vi "Write SSL Context.vi"(8 "error in (no error)":errorcluster, 10 "SSL_Lib.lvlib:SSL-Context.lvclass":refnum<class "SSL-Context.lvclass">, 11 "SSL Context in":refnum<class "SSL Context.lvclass">) -> (0 "error out":errorcluster, 3 "SSL Context out":refnum<class "SSL Context.lvclass">)   [LabVIEW 2013, in "OpenSSL Socket.lvlib" / "SSL Context.lvclass"]
uses:
  SSL Context.lvclass
  SSL_Lib/SSL-Context/SSL-Context.lvclass
  SSL Context.lvclass/SSL Context.ctl
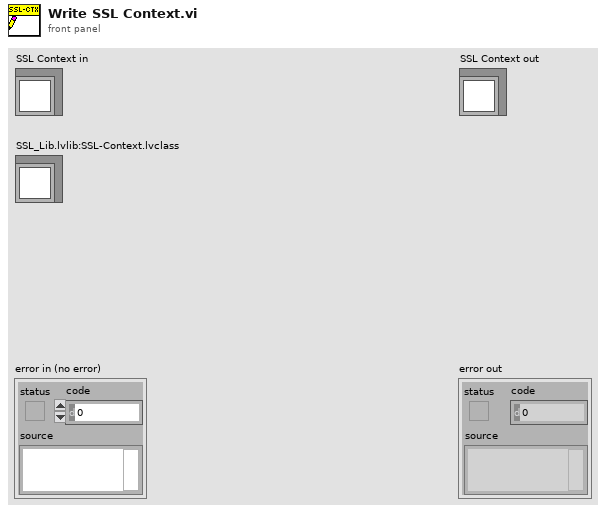
[diagram p1: front panel]
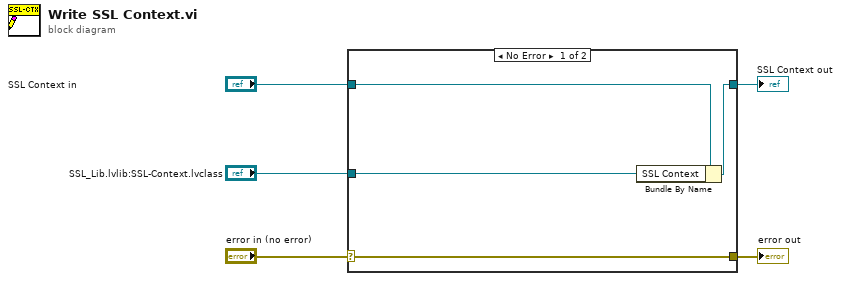
[diagram p0: block diagram]
diagram:
  n1 = case shown="No Error" "error in (no error)" {
    selector: "error in (no error)" -> [w9 w10]
    tunnel: [w9 w10] -> w4
    tunnel: [w7 w11] -> w2
    tunnel: "SSL Context in" -> [w8 w11]
    tunnel: "SSL_Lib.lvlib:SSL-Context.lvclass" -> [w6 _]
    frame No Error {
      n2 = Bundle By Name(cluster=w8, "SSL Context"=w6) -> (w7:refnum<class "SSL Context.lvclass">)
    }
    frame Error {
    }
  }
  "error out" <- w4
  "SSL Context out" <- w2
